vi "LabVIEW host computer v3.0.vi"() -> ()   [LabVIEW 2015]
uses:
  <vilib>/Instr/_visa.llb/VISA Configure Serial Port (Instr).vi
  <vilib>/Utility/file.llb/Read Delimited Spreadsheet (DBL).vi
  <vilib>/gmath/NI_Gmath.lvlib
panel:
  in  "选项卡控件":enum32{"双通道功率 ", "氢气浓度"}(tab)
  in  "选项卡控件 2":enum32{"通讯设置/数据显示"}(tab)
  in  "VISA resource name":refnum<visa-resource-name> caption="选择串口"
  in  "baud rate (9600)":u32=9600 caption="波特率"
  in  "氢气测量":bool
  out "CH1 Power":dbl
  out "?":string
  out "CH2 Power":dbl
  out "?":string
  out "CH1/CH2":dbl format="%#_3g"
  out "当前时间":string
  out "CH1 Power 2":dbl(graph)
  out "CH2 Power 2":dbl(graph)
  out "CH1/CH2  2":dbl(graph)
  out "氢气浓度":dbl[](graph)
  in  "氢气输入":dbl[](array[numeric])
  out "氢气变化波长":dbl
  out "氢气浓度 2":dbl
  out "标定X":dbl[](array[numeric])
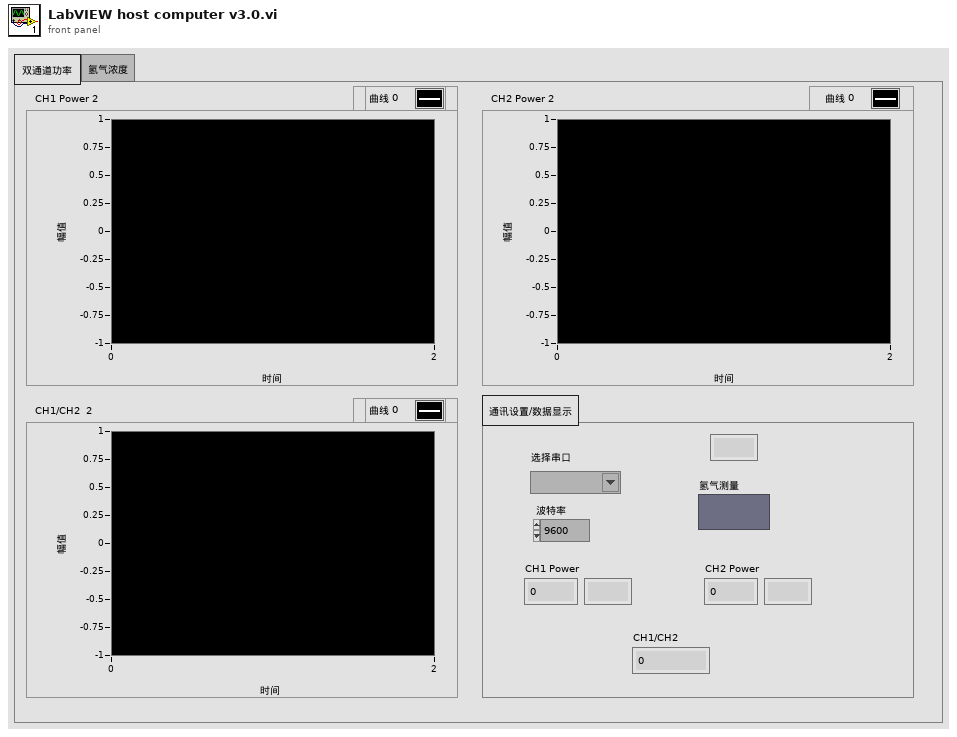
[diagram p1: front panel]
types:
  T1 = enum16{"open", "replace", "create", "open or create", "replace or create", "replace or create with confirmation"}
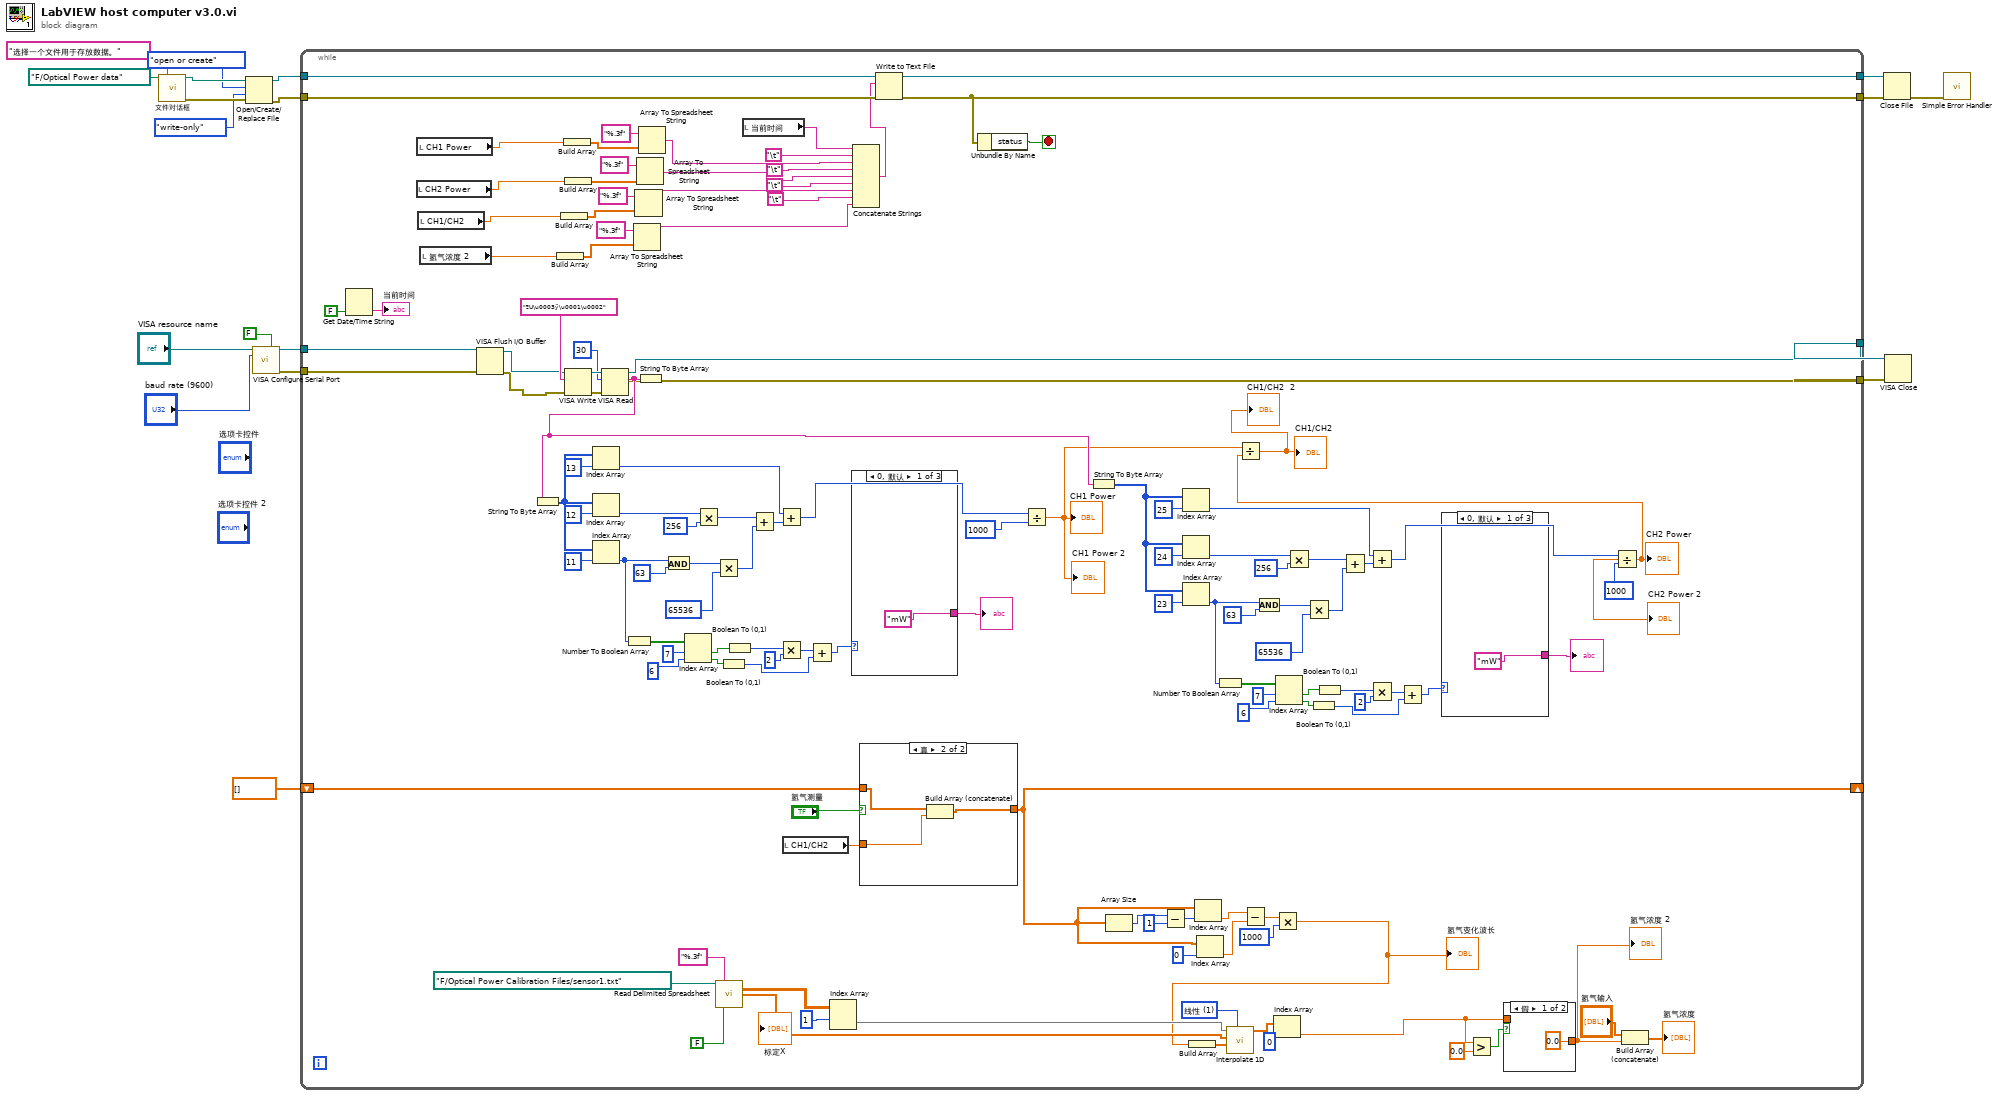
[diagram p0: block diagram]
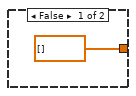
[diagram p3: hidden frame]
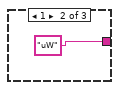
[diagram p4: hidden frame]
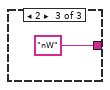
[diagram p5: hidden frame]
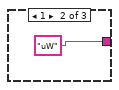
[diagram p6: hidden frame]
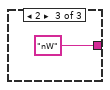
[diagram p7: hidden frame]
diagram:
  n1 = call "文件对话框"("start path"=path "F:/Optical Power data", "prompt"="选择一个文件用于存放数据。") -> ("selected path"=w9:path, "error out"=w8:errorcluster)  [unwired: 10 in, 2 out]
  n2 = Open/Create/Replace File(file path (use dialog)=w9, error in=w8, operation (0:open)=T1."open or create" ("操作(0:open)"), access (0:read/write)=enum16{"read/write", "read-only", "write-only"}."write-only" ("权限(0:read/write)")) -> (refnum out=w4:refnum<file>, error out=w5:errorcluster)  [unwired: 2 in, 1 out]
  n3 = call-poly "VISA Configure Serial Port"("VISA resource name"="VISA resource name", "Enable Termination\nChar (T)"=FALSE ("Enable Termination\nChar (T)"), "baud rate (9600)"="baud rate (9600)") -> ("VISA resource name out"=w16:refnum<visa-resource-name>, "error out"=w15:errorcluster)  [unwired: 11 in]
  n4 = while {
    tunnel: w16 -> [w85]
    tunnel: w15 -> [w84]
    tunnel: [w83] -> w14
    tunnel: [w80] -> w13
    shift-right: [w57] -> _
    shift-left: dbl[] [] -> [w61]
    tunnel: w5 -> [w52]
    tunnel: w4 -> [w51]
    tunnel: [w25] -> w2
    tunnel: [w27] -> w1
    stop <- w24 stop-if-true
    w67 = 1 items=["最近", "线性", "样条", "cubic Hermite", "拉格朗日"] ("method")
    n5 = Get Date/Time String(want seconds? (F)=FALSE ("需要秒？(F)")) -> (time string=→"当前时间":string)  [unwired: 2 in, 1 out]
    n6 = local read "CH2 Power"() -> (w49:dbl)
    n7 = local read "CH1 Power"() -> (w50:dbl)
    n8 = local read "CH1/CH2"() -> (w48:dbl)
    n9 = local read "氢气浓度 2"() -> (w47:dbl)
    n10 = VISA Flush I/O Buffer(VISA resource name=w85, error in (no error)=w84) -> (VISA resource name out=w115:refnum<visa-resource-name>, error out=w114:errorcluster)  [unwired: 1 in]
    n11 = Build Array(w47) -> (w30:dbl[])
    n12 = Build Array(w48) -> (w33:dbl[])
    n13 = Build Array(w50) -> (w38:dbl[])
    n14 = Build Array(w49) -> (w35:dbl[])
    n15 = VISA Write(VISA resource name=w115, write buffer="ªU\u0003ÿ\u0001\u0002" ("写入缓冲区"), error in (no error)=w114) -> (VISA resource name out=w145:refnum<visa-resource-name>, error out=w144:errorcluster)  [unwired: 1 out]
    n16 = VISA Read(VISA resource name=w145, byte count=u32 30 ("字节总数"), error in (no error)=w144) -> (VISA resource name out=w83:refnum<visa-resource-name>, read buffer=w86:string, error out=w80:errorcluster)  [unwired: 1 out]
    n17 = String To Byte Array(string=w86) -> (unsigned byte array=w141:u8[])
    n18 = Index Array(array=w141, index=13) -> (element=w126:u8)
    n19 = Index Array(array=w141, index=12) -> (element=w132:u8)
    n20 = Index Array(array=w141, index=11) -> (element=w138:u8)
    n21 = Number To Boolean Array(number=w138) -> (Boolean array=w139:bool[])
    n22 = Array To Spreadsheet String(array=w30, 3:"%.3f" ("格式字符串")) -> (spreadsheet string=w28:string)  [unwired: 1 in]
    n23 = Array To Spreadsheet String(array=w33, 3:"%.3f" ("格式字符串")) -> (spreadsheet string=w31:string)  [unwired: 1 in]
    n24 = Array To Spreadsheet String(array=w35, 3:"%.3f" ("格式字符串")) -> (spreadsheet string=w34:string)  [unwired: 1 in]
    n25 = String To Byte Array(string=w86) -> ()  [unwired: 1 out]
    n26 = Array To Spreadsheet String(array=w38, 3:"%.3f" ("格式字符串")) -> (spreadsheet string=w37:string)  [unwired: 1 in]
    n27 = And(x=w138, y=63) -> (x .and. y?=w130:i32)
    n28 = Index Array(array=w139, index #1=7 ("index"), index #2=6 ("索引")) -> (element #1=w124:bool, element #2=w122:bool)
    n29 = Multiply(x=w132, y=u32 256) -> (x*y=w134:u32)
    n30 = Multiply(x=w130, y=u32 65536) -> (x*y=w135:u32)
    n31 = call-poly <vilib>:"Read Delimited Spreadsheet.vi"("file path (dialog if empty)"=path "F:/Optical Power Calibration Files/sensor1.txt" ("基路径"), "format (%.3f)"="%.3f", "transpose? (F)"=FALSE ("transpose (no:F)")) -> ("all rows"=w72:dbl[][], "first row"=w64:dbl[])  [unwired: 7 in, 4 out]
    "标定X" <- w64
    n32 = Boolean To (0,1)(Boolean=w122) -> (0, 1=w119:i16)
    n33 = Boolean To (0,1)(Boolean=w124) -> (0, 1=w123:i16)
    n34 = local read "当前时间"() -> (w42:string)
    n35 = Add(x=w134, y=w135) -> (x+y=w136:u32)
    n36 = Add(x=w126, y=w136) -> (x+y=w117:u32)
    n37 = Multiply(x=w123, y=2 ("index")) -> (x*y=w120:i32)
    n38 = local read "CH1/CH2"() -> (w22:dbl)
    n39 = Add(x=w120, y=w119) -> (x+y=w118:i32)
    n40 = Index Array(array=w72, index (row)=1 ("索引 (行)")) -> (element=w65:dbl[])  [unwired: 1 in]
    n41 = case shown="0, 默认" w118 {
      tunnel: ["mW" "uW" "nW"] -> w116
      frame 0, Default {
      }
      frame 1 {
      }
      frame 2 {
      }
    }
    "?" <- w116
    n42 = Concatenate Strings(w42, "\t", w37, "\t", w34, "\t", w31, "\t", w28) -> (w26:string)
    n43 = case shown="真" "氢气测量" {
      tunnel: [dbl[] [] w152] -> w57
      tunnel: w61 -> [_ w151]
      tunnel: w22 -> [_ w150]
      frame False {
      }
      frame True {
        n44 = Build Array (concatenate)(w151, w150) -> (w152:dbl[])
      }
    }
    n45 = Write to Text File(file (use dialog)=w51, text=w26, error in=w52) -> (refnum out=w27:refnum<file>, error out=w25:errorcluster)  [unwired: 1 in, 1 out]
    n46 = Unbundle By Name(w25) -> ("status"=w24:bool)
    n47 = Divide(x=w117, y=u32 1000) -> (x/y=w82:dbl)
    "CH1 Power" <- w82
    "CH1 Power 2" <- w82
    n48 = String To Byte Array(string=w86) -> (unsigned byte array=w112:u8[])
    n49 = Array Size(array=w57) -> (size(s)=w77:i32)
    n50 = Subtract(x=w77, y=1) -> (x-y=w78:i32)
    n51 = Index Array(array=w112, index=25) -> (element=w97:u8)
    n52 = Index Array(array=w112, index=24) -> (element=w103:u8)
    n53 = Index Array(array=w112, index=23) -> (element=w109:u8)
    n54 = Index Array(array=w57, index=w78) -> (element=w60:dbl)
    n55 = Index Array(array=w57, index=0 ("y")) -> (element=w59:dbl)
    n56 = Number To Boolean Array(number=w109) -> (Boolean array=w110:bool[])
    n57 = Subtract(x=w60, y=w59) -> (x-y=w74:dbl)
    n58 = And(x=w109, y=63) -> (x .and. y?=w101:i32)
    n59 = Multiply(x=w74, y=1000) -> (x*y=w55:dbl)
    "氢气变化波长" <- w55
    n60 = Build Array(w55) -> (w66:dbl[])
    n61 = call <vilib>:"Interpolate 1D.vi"("method"=w67, "xi"=w66, "X"=w64, "Y"=w65) -> ("yi"=w68:dbl[])  [unwired: 5 in, 2 out]
    n62 = Index Array(array=w68, index=0 ("索引")) -> (element=w58:dbl)
    n63 = Index Array(array=w110, index #1=7 ("index"), index #2=6 ("索引")) -> (element #1=w95:bool, element #2=w93:bool)
    n64 = Multiply(x=w103, y=u32 256) -> (x*y=w105:u32)
    n65 = Multiply(x=w101, y=u32 65536) -> (x*y=w106:u32)
    n66 = Boolean To (0,1)(Boolean=w93) -> (0, 1=w90:i16)
    n67 = Boolean To (0,1)(Boolean=w95) -> (0, 1=w94:i16)
    n68 = Add(x=w105, y=w106) -> (x+y=w107:u32)
    n69 = Add(x=w97, y=w107) -> (x+y=w88:u32)
    n70 = Multiply(x=w94, y=2 ("index")) -> (x*y=w91:i32)
    n71 = Add(x=w91, y=w90) -> (x+y=w89:i32)
    n72 = case shown="0, 默认" w89 {
      tunnel: ["mW" "uW" "nW"] -> w87
      frame 0, Default {
      }
      frame 1 {
      }
      frame 2 {
      }
    }
    "?" <- w87
    n73 = Greater?(x=w58, y=0.0) -> (0:w63:bool)
    n74 = case shown="假" w63 {
      tunnel: w58 -> [_ w148]
      tunnel: [0.0 ("Numeric") w148] -> w54
      frame False {
      }
      frame True {
      }
    }
    "氢气浓度 2" <- w54
    n75 = Divide(x=w88, y=u32 1000) -> (x/y=w81:dbl)
    "CH2 Power" <- w81
    "CH2 Power 2" <- w81
    n76 = Divide(x=w82, y=w81) -> (x/y=→"CH1/CH2" →"CH1/CH2  2":dbl)
    n77 = Build Array (concatenate)("氢气输入", w54) -> (→"氢气浓度":dbl[])
  }
  n78 = Close File(refnum=w1, error in=w2) -> (error out=w3:errorcluster)  [unwired: 1 out]
  n79 = VISA Close(VISA resource name=w14, error in (no error)=w13) -> ()  [unwired: 1 out]
  n80 = call <vilib>:"Simple Error Handler.vi"("error in (no error)"=w3) -> ()  [unwired: 4 in, 5 out]
